vi "Write ItemObjs.vi"(10 "ItemObjs":refnum<class "BetterItem.lvclass">[](array[class]), 11 "BetterHandle in":refnum<class "BetterHandle.lvclass">) -> (3 "BetterHandle out":refnum<class "BetterHandle.lvclass">)   [LabVIEW 2020, in "BetterDragAndDrop.lvlib" / "BetterHandle.lvclass"]
uses:
  BetterHandle.lvclass
  BetterTreeItem/BetterItem.lvclass
  BetterHandle.lvclass/BetterHandle.ctl
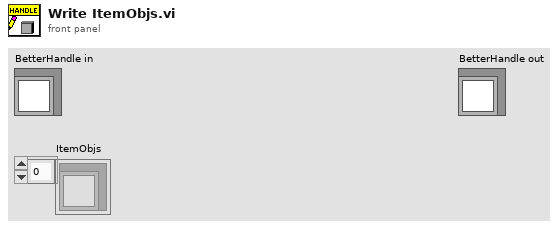
[diagram p1: front panel]
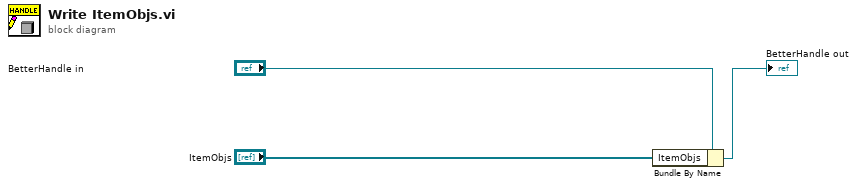
[diagram p0: block diagram]
diagram:
  n1 = Bundle By Name(cluster="BetterHandle in", "ItemObjs"="ItemObjs") -> (→"BetterHandle out":refnum<class "BetterHandle.lvclass">)
